vi "Operation UI.vi"(0 "A":dbl, 5 "B":dbl, 7 "Calculate":bool, 9 "DVR In":refnum<data-value>, 11 "Error In":errorcluster) -> (4 "C":dbl, 10 "DVR  Out":refnum<data-value>, 15 "Error Out":errorcluster)   [LabVIEW 2023, in "Divide.lvclass"]
doc: "The VI contains the addition operation UI that accepts two input numbers and performs division operation and displays the output when user clicks calculate button"
uses:
  Divide.lvclass
  Arithemtic Operation/Arithemetic Operation.lvclass
  Typedef/User Event Operations.ctl
panel:
  # "DIVISION"
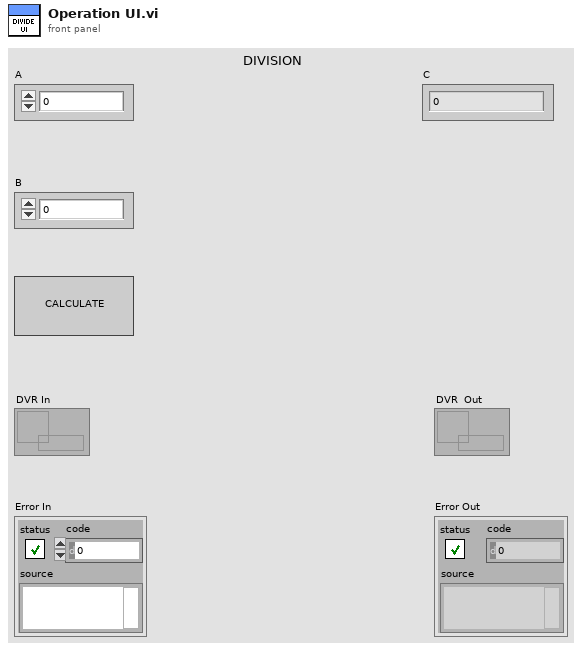
[diagram p1: front panel]
types:
  T1 = typedef "User Event Operations.ctl" = enum16{"Obtain", "Generate", "Destroy"}
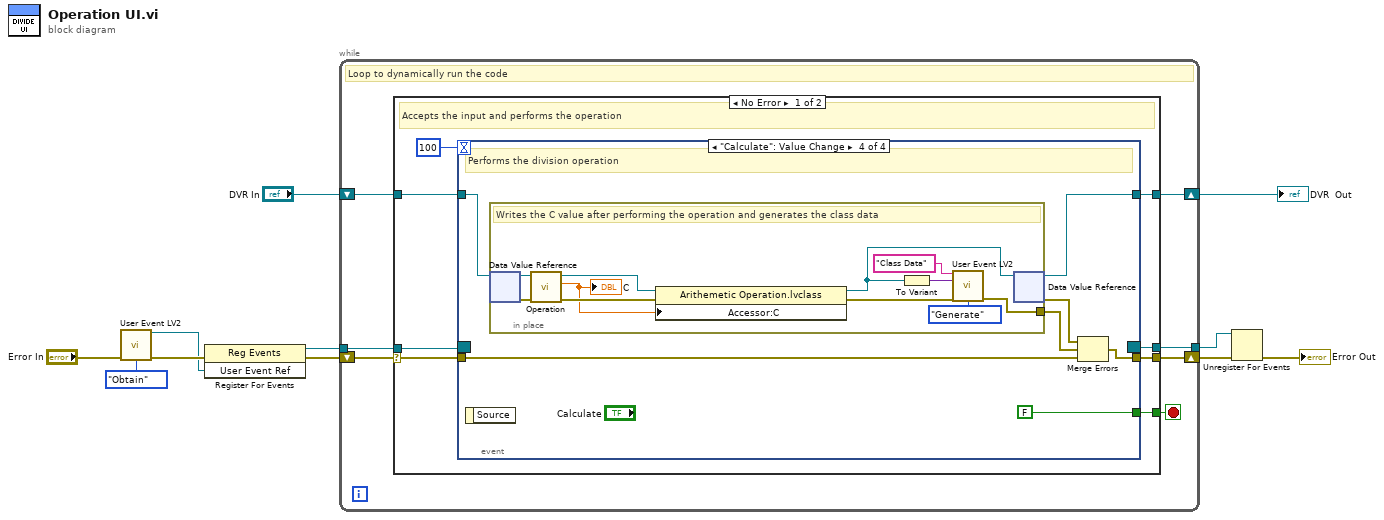
[diagram p0: block diagram]
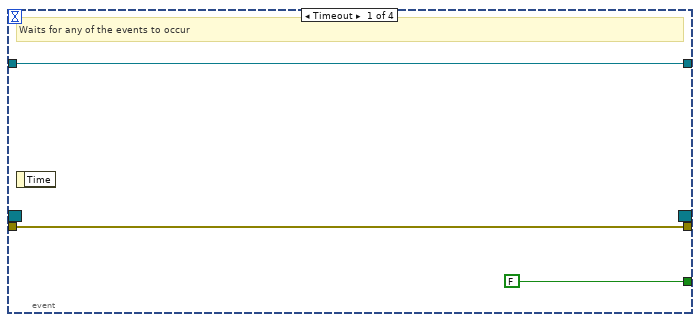
[diagram p2: hidden frame]
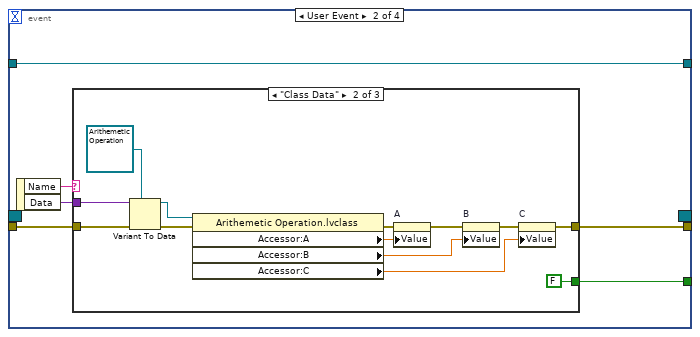
[diagram p3: hidden frame]
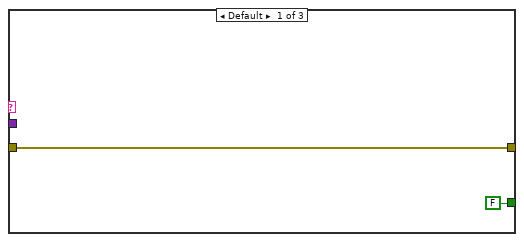
[diagram p4: hidden frame]
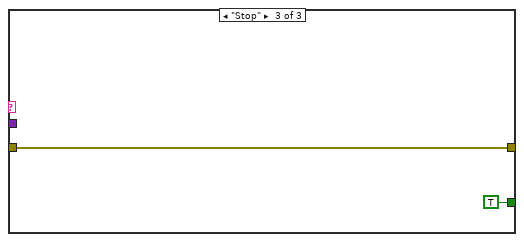
[diagram p5: hidden frame]
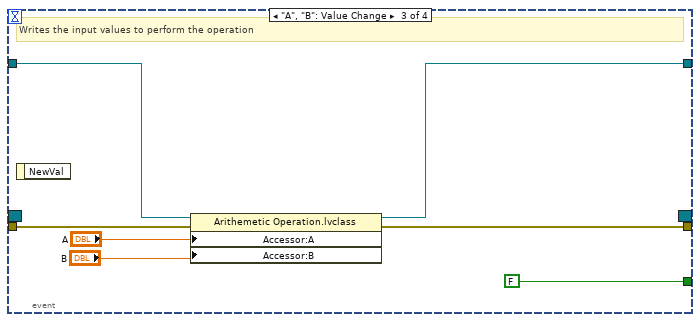
[diagram p6: hidden frame]
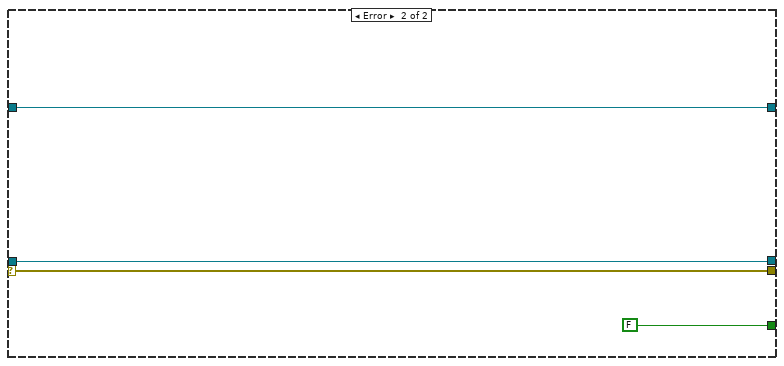
[diagram p7: hidden frame]
diagram:
  n1 = call "User Event LV2.vi"("Error In"="Error In", "Operation"=User_Event_Operations."Obtain") -> ("User Event Ref"=w1:refnum<user-event>, "Error Out"=w3:errorcluster)  [unwired: 12 in]
  n2 = register-events(error in=w3, w1) -> (reference out=w8:refnum<event-registration>, error out=w9:errorcluster)  [unwired: 1 in]
  n3 = while {
    shift-right: [w17] -> w11
    shift-left: w9 -> [w18]
    shift-right: [w15] -> w4
    shift-left: "DVR In" -> [w16]
    tunnel: w8 -> [w14]
    tunnel: [w13] -> w6
    stop <- w12 stop-if-true
    # "Loop to dynamically run the code"
    n4 = case shown="No Error" w18 {
      selector: w18 -> [w24 w81]
      tunnel: [w23 w81] -> w17
      tunnel: [w25 w80] -> w15
      tunnel: w16 -> [w26 w80]
      tunnel: w14 -> [w21 w79]
      tunnel: [w20 w79] -> w13
      tunnel: [w19 FALSE] -> w12
      frame No Error {
        # "Accepts the input and performs the operation"
        n5 = event shown="[3] \"Calculate\": Value Change" {
          selector: w21 -> [_ _ _ _]
          dyn-events: [_ _ _ _] -> w20
          timeout: 100 -> [_ _ _ _]
          tunnel: [w29 w35 w54 w64] -> w25
          tunnel: w26 -> [w29 w35 w57 w65]
          tunnel: w24 -> [w28 w34 w59 w60]
          tunnel: [w28 w32 w58 w63] -> w23
          tunnel: [FALSE w30 FALSE FALSE] -> w19
          event Timeout {
            # "Waits for any of the events to occur"
            n6 = event-data() -> ()  [unwired: 1 in, 1 out]
          }
          event User Event {
            n7 = event-data() -> ("Name"=w33:string, "Data"=w31:variant)  [unwired: 1 in]
            n8 = case shown="\"Class Data\"" w33 {
              tunnel: w34 -> [w37 w50 w52]
              tunnel: [w37 w46 w52] -> w32
              tunnel: w31 -> [_ w41 _]
              tunnel: [FALSE FALSE TRUE] -> w30
              frame Default {
              }
              frame "Class Data" {
                n9 = Variant To Data(error in=w50, type=refnum<class "Arithemetic Operation.lvclass"> refnum ("reference"), Variant=w41) -> (data=w40:refnum<class "Arithemetic Operation.lvclass">, error out=w42:errorcluster)
                n10 = property class="Arithemetic Operation.lvclass"(reference=w40, error in=w42) -> (error out=w49:errorcluster, "Accessor:A"=w45:dbl, "Accessor:B"=w44:dbl, "Accessor:C"=w43:dbl)  [unwired: 1 out]
                n11 = property on="A" class="DigNum (strict)"(error in=w49, "Value"=w45) -> (error out=w48:errorcluster)  [unwired: 1 in, 1 out]
                n12 = property on="B" class="DigNum (strict)"(error in=w48, "Value"=w44) -> (error out=w47:errorcluster)  [unwired: 1 in, 1 out]
                n13 = property on="C" class="DigNum (strict)"(error in=w47, "Value"=w43) -> (error out=w46:errorcluster)  [unwired: 1 in, 1 out]
              }
              frame "Stop" {
              }
            }
          }
          event "A", "B": Value Change {
            # "Writes the input values to perform the operation"
            n14 = event-data() -> ()  [unwired: 1 in, 1 out]
            n15 = property class="Arithemetic Operation.lvclass"(reference=w57, error in=w59, "Accessor:A"="A", "Accessor:B"="B") -> (reference out=w54:refnum<data-value>, error out=w58:errorcluster)
          }
          event "Calculate": Value Change {
            # "Performs the division operation"
            n16 = event-data() -> ()  [unwired: 1 in, 1 out]
            n17 = in-place {
              in-place-border: [w70] -> w61
              # "Writes the C value after performing the operation and generates the class data"
              n18 = in-place-dvr #1(w65) -> (w74:refnum<class "Arithemetic Operation.lvclass">, w73:errorcluster)
              n19 = call-dynamic "Operation.vi"("Error In"=w73, "Arithemetic Operation in"=w74) -> ("Error Out"=w77:errorcluster, "C"=w75:dbl, "Arithemetic Operation out"=w76:refnum<class "Arithemetic Operation.lvclass">)  [unwired: 7 in]
              "C" <- w75
              n20 = property class="Arithemetic Operation.lvclass"(reference=w76, error in=w77, "Accessor:C"=w75) -> (reference out=w68:refnum<class "Arithemetic Operation.lvclass">, error out=w69:errorcluster)
              n21 = To Variant(anything=w68) -> (Variant=w72:variant)
              n22 = call "User Event LV2.vi"("Event Name"="Class Data", "Data"=w72, "Error In"=w69, "Operation"=User_Event_Operations."Generate") -> ("Error Out"=w70:errorcluster)  [unwired: 10 in, 1 out]
              n23 = in-place-dvr #1(w68) -> (w64:refnum<data-value>, w62:errorcluster)
            }
            n24 = Merge Errors(w62, w61, w60) -> (w63:errorcluster)
          }
        }
      }
      frame Error {
      }
    }
  }
  "DVR  Out" <- w4
  n25 = Unregister For Events(event registration refnum=w6, error in=w11) -> (error out=→"Error Out":errorcluster)
